vi "Handle Dynamic VI call errors.vi"(3 "error in (no error)":errorcluster) -> (1 "error out":errorcluster)   [LabVIEW 2016, in "Nanonis Prog Interface.lvlib"]
uses:
  Nanonis Prog Interface.lvlib
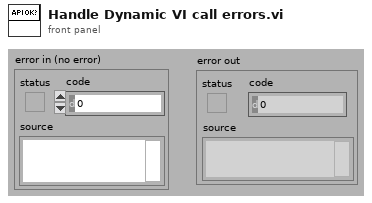
[diagram p1: front panel]
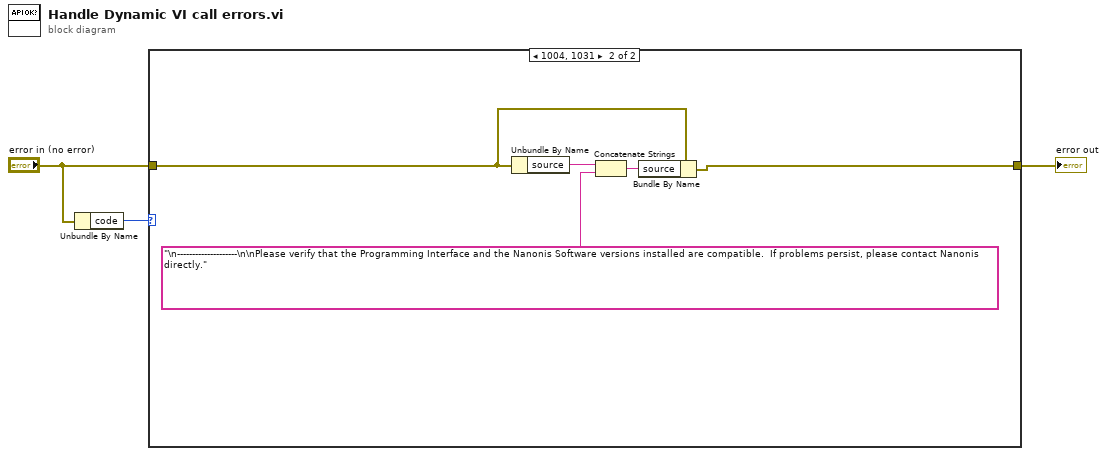
[diagram p0: block diagram]
diagram:
  n1 = Unbundle By Name("error in (no error)") -> ("code"=w3:i32)
  n2 = case shown="1004, 1031" w3 {
    tunnel: "error in (no error)" -> [w4 w7]
    tunnel: [w4 w5] -> w1
    frame 0, Default {
    }
    frame 1004, 1031 {
      n3 = Unbundle By Name(w7) -> ("source"=w9:string)
      n4 = Concatenate Strings(w9, "\n--------------------\n\nPlease verify that the Programming Interface and the Nanonis Software versions installed are compatible.  If problems persist, please contact Nanonis directly.") -> (w6:string)
      n5 = Bundle By Name(cluster=w7, "source"=w6) -> (w5:errorcluster)
    }
  }
  "error out" <- w1
